vi "TCP File Sender.vi"() -> ()   [LabVIEW 2015]
doc: "This VI supports a TCP file transfer application. Data is read from an FPGA personality, stored to a spreadsheet file, then transfered via TCP. The TCP File Receiver.vi will then collect the spreadsheet file and format the data for display."
uses:
  <vilib>/FPGAPlugInAG/sbRIO-9637/niLvFpga_Open_sbRIO-9637.vi
  <vilib>/rvi/interface/common/dynamic/niFpgaDynamicAddResources.vi
  <vilib>/Utility/error.llb/Error Cluster From Error Code.vi
  <vilib>/rvi/errors/niLvFpgaAdjustHostInterfaceError.vi
  <vilib>/Utility/file.llb/Write Delimited Spreadsheet (DBL).vi
  <vilib>/rvi/interface/nirviOpenFPGA/nirviOpenFPGA.xnode
  FPGA Bitfiles/TCPFileTransfer-_FPGATarget_FPGAPersonality_kgR9C5aWxQc.lvbitx
  <vilib>/rvi/interface/nirviMethod/nirviMethod.xnode
  <vilib>/FPGAPlugInAG/Dynamic/niLvFpga_ReadFifo_Dynamic.vi
  <vilib>/rvi/errors/niLvFpgaMergeErrorWithErrorCode.vi
panel:
  in  "RTOS File Path":path=path "C:/ni-rt/Waveform Data.dat"
  in  "Port":u16=5280
  in  "Host PC\nAddress":string="172.22.11.1"
  in  "Chunk Size":i32=1000
  # "In this application, sine wave data is read from the FPGA, stored to a spreadsheet file, then \ntransfered via TCP in chunks. The TCP File Receiver.vi, running on your PC, will then collect\nthe spreadsheet file and format the data for display. Specify the IP address of your host \nPC in the 'Host PC Address' control below; 172.22.11.1 is the default if using USB connection."
  # "Alternatively, you can login to your target and read the unformatted file in your browser. Open NI MAX (Measurement and Automation Explorer) and right-click on your eval kit under Remote Systems, then select File Transfer. You will be prompted to login to the target, where the default credentials are 'admin' and 'blank'. Then you can navigate the target's file directory to the path you indicated in the RTOS File Path control above.\n\nIf connected over USB and using the default RTOS File Path above, the default browser location to view your file is:\nhttp://172.22.11.2/files/C/ni-rt/Waveform%20Data.dat"
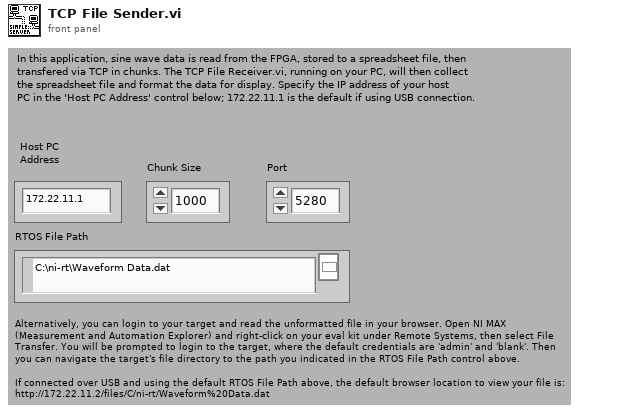
[diagram p1: front panel]
types:
  T1 = enum16{"open", "replace", "create", "open or create", "replace or create", "replace or create with confirmation"}
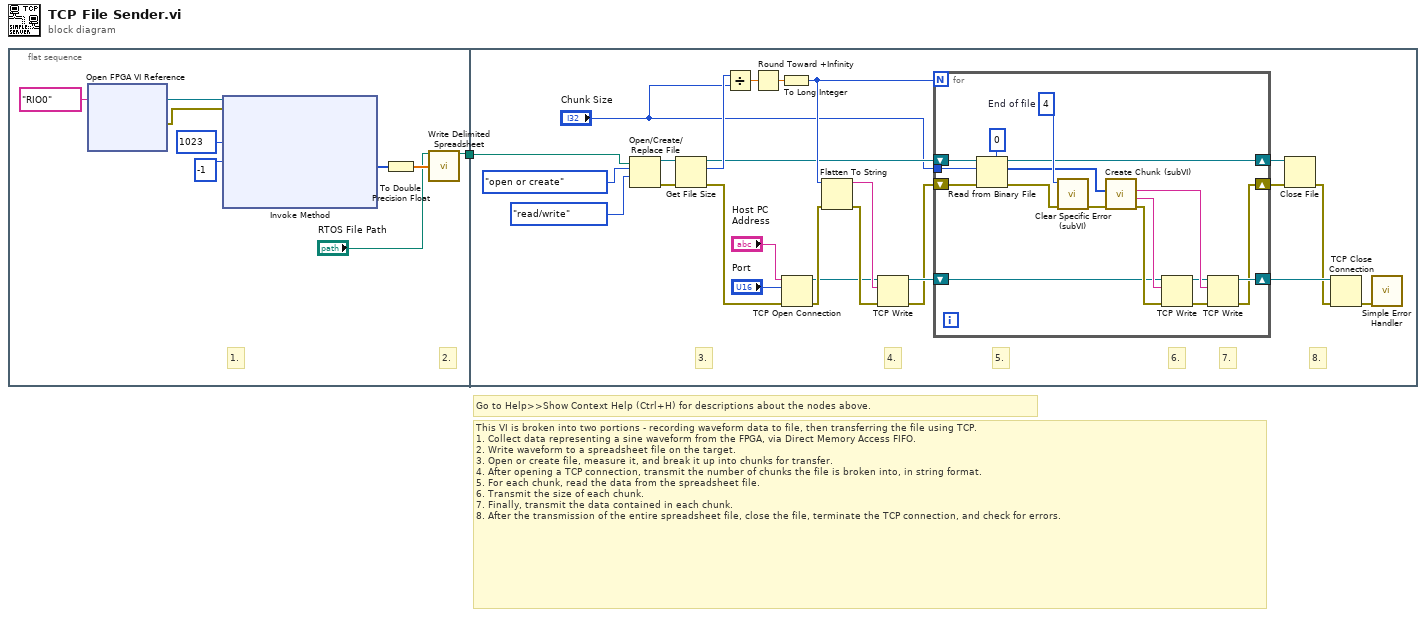
[diagram p0: block diagram]
diagram:
  # "Go to Help>>Show Context Help (Ctrl+H) for descriptions about the nodes above."
  # "This VI is broken into two portions - recording waveform data to file, then transferring the file using TCP.\n1. Collect data representing a sine waveform from the FPGA, via Direct Memory Access FIFO.\n2. Write waveform to a spreadsheet file on the target.\n3. Open or create file, measure it, and break it up into chunks for transfer.  \n4. After opening a TCP connection, transmit the number of chunks the file is broken into, in string format.\n5. For each chunk, read the data from the spreadsheet file.\n6. Transmit the size of each chunk.\n7. Finally, transmit the data contained in each chunk.\n8. After the transmission of the entire spreadsheet file, close the file, terminate the TCP connection, and check for errors."
  n1 = flat-sequence {
    tunnel: [w5] -> w1
    tunnel: w1 -> [w11]
    frame #0 {
      # "2."
      # "1."
      n2 = xnode "Open FPGA VI Reference"("resource name"=tag "RIO0") -> ("FPGA VI Reference Out"=w4:refnum<k20>, "error out"=w3:errorcluster)  [unwired: 1 in]
      n3 = xnode "Invoke Method"("FPGA VI Reference In"=w4, "error in"=w3, "Number of Elements"=u32 1023, "Timeout (ms)"=-1) -> ("Data"=w8:i16[])  [unwired: 3 out]
      n4 = To Double Precision Float(number=w8) -> (double precision float=w7:dbl[])
      n5 = call-poly <vilib>:"Write Delimited Spreadsheet.vi"("file path (dialog if empty)"="RTOS File Path", "1D data"=w7) -> ("new file path (Not A Path if cancelled)"=w5:path)  [unwired: 12 in, 1 out]
    }
    frame #1 {
      # "7."
      # "6."
      # "5."
      # "8."
      # "4."
      # "3."
      n6 = Open/Create/Replace File(file path (use dialog)=w11, operation (0:open)=T1."open or create", access (0:read/write)=enum16{"read/write", "read-only", "write-only"}."read/write") -> (refnum out=w23:refnum<file>, error out=w31:errorcluster)  [unwired: 1 in, 3 out]
      n7 = Get File Size(file=w23, error in=w31) -> (refnum out=w18:refnum<file>, size (in bytes)=w27:i64, 0:w30:errorcluster)
      n8 = Divide(x=w27, y="Chunk Size") -> (x/y=w28:dbl)
      n9 = Round Toward +Infinity(x=w28) -> (ceil(x): smallest int >= x=w29:dbl)
      n10 = To Long Integer(number=w29) -> (32bit integer=w21:i32)
      n11 = TCP Open Connection(address="Host PC\nAddress", remote port or service name="Port", error in (no error)=w30) -> (connection ID=w22:refnum<k5>, error out=w25:errorcluster)  [unwired: 1 in, 1 out]
      n12 = Flatten To String(anything=w21, error in (no error)=w25) -> (data string=w26:string, error out=w24:errorcluster)  [unwired: 3 out]
      n13 = TCP Write(connection ID=w22, data in=w26, error in (no error)=w24) -> (connection ID out=w20:refnum<k5>, error out=w19:errorcluster)  [unwired: 2 out]
      n14 = for {
        N: w21 -> [_]
        shift-right: [w46] -> w16
        shift-left: w18 -> [w50]
        shift-right: [w36] -> w15
        shift-left: w19 -> [w49]
        shift-right: [w37] -> w14
        shift-left: w20 -> [w39]
        tunnel: "Chunk Size" -> [w45]
        w51 = 4  # End of file
        n15 = Read from Binary File(5:u8 0, 8:w49, 10:w45, 11:w50) -> (0:w48:errorcluster, 2:w44:u8[], 3:w46:refnum<file>)  [unwired: 3 out]
        n16 = call "Clear Specific Error (subVI).vi"("error in (no error)"=w48, "Code"=w51) -> ("error out"=w47:errorcluster)  [unwired: 5 out]
        n17 = call "Create Chunk (subVI).vi"("error in (no error)"=w47, "Byte Array"=w44) -> ("error out"=w41:errorcluster, "size string"=w43:string, "Chunk String"=w42:string)  [unwired: 7 out]
        n18 = TCP Write(connection ID=w39, data in=w43, error in (no error)=w41) -> (connection ID out=w38:refnum<k5>, error out=w40:errorcluster)  [unwired: 2 out]
        n19 = TCP Write(connection ID=w38, data in=w42, error in (no error)=w40) -> (connection ID out=w37:refnum<k5>, error out=w36:errorcluster)  [unwired: 2 out]
      }
      n20 = Close File(refnum=w16, error in=w15) -> (error out=w13:errorcluster)  [unwired: 1 out]
      n21 = TCP Close Connection(connection ID=w14, error in (no error)=w13) -> (error out=w12:errorcluster)  [unwired: 2 out]
      n22 = call <vilib>:"Simple Error Handler.vi"("error in (no error)"=w12) -> ()  [unwired: 1 in, 8 out]
    }
  }
